vi "Write Card Array.vi"(8 "error in (no error)":errorcluster, 10 "Value":bool[](array[boolean]), 11 "Universal Power Meter.lvlib:Universal Power Meter.lvclass":refnum<class "Universal Power Meter.lvclass">) -> (0 "error out":errorcluster, 3 "Universal Power Meter out":refnum<class "Universal Power Meter.lvclass">)   [LabVIEW 2014, in "Universal Power Meter.lvlib" / "Universal Power Meter.lvclass"]
uses:
  Universal Power Meter.lvclass
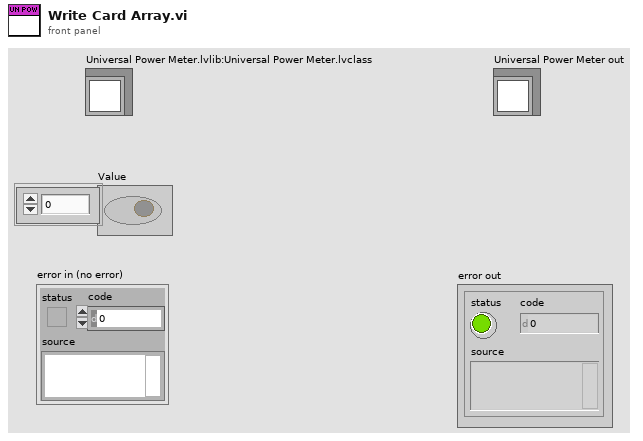
[diagram p1: front panel]
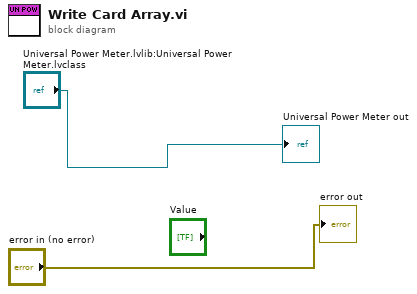
[diagram p0: block diagram]
diagram:
  "Universal Power Meter out" <- "Universal Power Meter.lvlib:Universal Power Meter.lvclass"
  "error out" <- "error in (no error)"
